vi "SetParameter.vi"(1 "Comment":string, 2 "Value":string, 3 "Parameter":string) -> (0 "Error":bool)   [LabVIEW 2014]
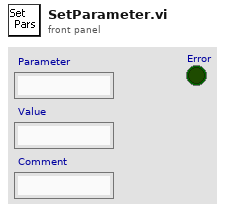
[diagram p1: front panel]
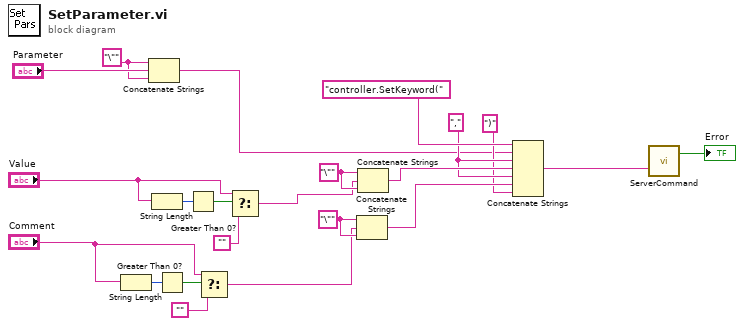
[diagram p0: block diagram]
diagram:
  w2 = "\"" ("string")
  w5 = "," ("string")
  w16 = "\"" ("string")
  w17 = "\"" ("string")
  n1 = String Length(string="Comment") -> (length=w15:i32)
  n2 = Concatenate Strings(w2, "Parameter", w2) -> (w1:string)
  n3 = String Length(string="Value") -> (length=w11:i32)
  n4 = Greater Than 0?(x=w15) -> (x > 0?=w14:bool)
  n5 = Greater Than 0?(x=w11) -> (x > 0?=w12:bool)
  n6 = Select(t="Comment", s=w14, f="") -> (s? t:f=w13:string)
  n7 = Select(t="Value", s=w12, f="") -> (s? t:f=w10:string)
  n8 = Concatenate Strings(w16, w13, w16) -> (w4:string)
  n9 = Concatenate Strings(w17, w10, w17) -> (w7:string)
  n10 = Concatenate Strings("controller.SetKeyword(" ("string"), w1, w5, w7, w5, w4, ")" ("string")) -> (w20:string)
  n11 = call "ServerCommand.vi"("Command"=w20) -> ("Error"=→"Error":bool)  [unwired: 1 out]
